vi "edittest read test steps from file.vi"(8 "error in (no error)":errorcluster, 9 "Version":string, 11 "File Refnum In":T2) -> (0 "error out":errorcluster, 2 "Sequence Steps":T1[](array[typedef]), 3 "File Refnum Out":T2)   [LabVIEW 2011]
uses:
  <vilib>/Utility/config.llb/Config Data RefNum.ctl
  server/database/Steps/Step Record.ctl
  <vilib>/Utility/config.llb/Read Key (I32).vi
  <vilib>/Utility/config.llb/Read Key (String).vi
  <vilib>/Utility/config.llb/NI_LVConfig.lvlib
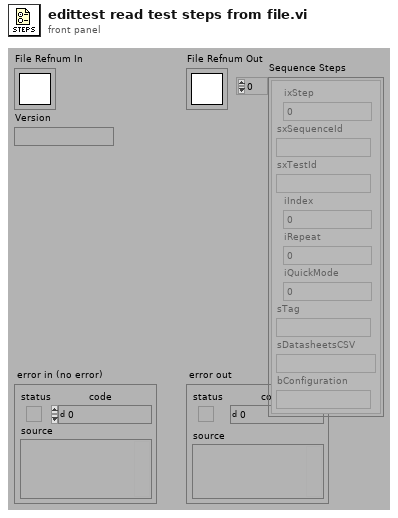
[diagram p1: front panel]
types:
  T1 = typedef "Step Record.ctl" = cluster{"ixStep":i32, "sxSequenceId":string, "sxTestId":string, "iIndex":i32, "iRepeat":i32, "iQuickMode":i32, "sTag":string, "sDatasheetsCSV":string, "bConfiguration":string}
  T2 = typedef "NI_LVConfig.lvlib/Config Data RefNum.ctl" = refnum<k1>
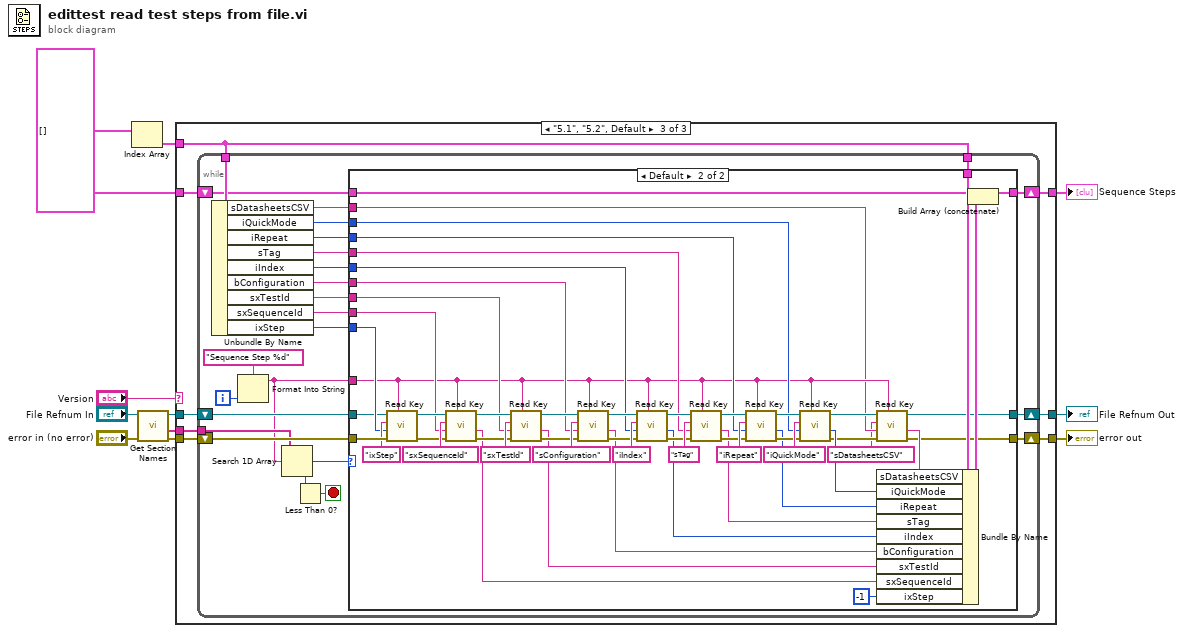
[diagram p0: block diagram]
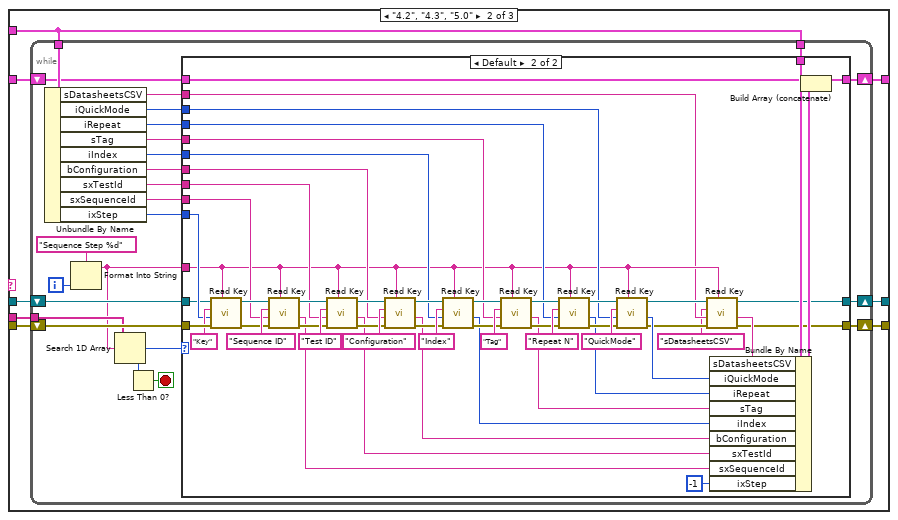
[diagram p3: hidden frame]
diagram:
  w3 = T1[] []
  n1 = Index Array(array=w3) -> (element=w4:T1)  [unwired: 1 in]
  n2 = call <vilib>:"Get Section Names.vi"("error in (no error)"="error in (no error)", "refnum"="File Refnum In") -> ("error out"=w7:errorcluster, "section names"=w5:string[], "refnum out"=w6:T2)  [unwired: 7 out]
  n3 = case shown="\"5.1\", \"5.2\", Default" "Version" {
    tunnel: [w12 w21 w107] -> w11
    tunnel: [w13 w20 w106] -> w10
    tunnel: w7 -> [w12 w19 w105]
    tunnel: w6 -> [w13 w18 w104]
    tunnel: w5 -> [_ w17 w103]
    tunnel: w4 -> [_ w16 w102]
    tunnel: w3 -> [_ w15 w101]
    tunnel: [_ w14 w100] -> w2
    frame "-1.0" {
    }
    frame "4.2", "4.3", "5.0" {
      n4 = while {
        shift-right: [w40] -> w20
        shift-left: w18 -> [w28]
        shift-right: [w41] -> w21
        shift-left: w19 -> [w42]
        tunnel: w16 -> [w39]
        tunnel: w16 -> [w30]
        tunnel: w17 -> [w27]
        shift-right: [w22] -> w14
        shift-left: w15 -> [w23]
        i -> [w43]
        stop <- w24 stop-if-true
        n5 = Unbundle By Name(w39) -> ("sDatasheetsCSV"=w29:string, "iQuickMode"=w31:i32, "iRepeat"=w32:i32, "sTag"=w33:string, "iIndex"=w34:i32, "bConfiguration"=w35:string, "sxTestId"=w36:string, "sxSequenceId"=w37:string, "ixStep"=w38:i32)
        n6 = Format Into String(format string="Sequence Step %d", w43) -> (resulting string=w26:string)  [unwired: 2 in, 1 out]
        n7 = Search 1D Array(1D array=w27, element=w26) -> (index of element=w25:i32)  [unwired: 1 out]
        n8 = Less Than 0?(x=w25) -> (x < 0?=w24:bool)
        n9 = case shown="Default" w25 {
          tunnel: w42 -> [w47 w99]
          tunnel: w26 -> [_ w54]
          tunnel: [w47 w49] -> w41
          tunnel: [w46 w48] -> w40
          tunnel: w38 -> [_ w76]
          tunnel: w37 -> [_ w75]
          tunnel: w36 -> [_ w74]
          tunnel: w35 -> [_ w73]
          tunnel: w34 -> [_ w72]
          tunnel: w33 -> [_ w71]
          tunnel: w32 -> [_ w70]
          tunnel: w31 -> [_ w69]
          tunnel: w30 -> [_ w68]
          tunnel: w29 -> [_ w52]
          tunnel: w28 -> [w46 w60]
          tunnel: w23 -> [w45 w59]
          tunnel: [w45 w57] -> w22
          frame -1 {
          }
          frame Default {
            n10 = call-poly <vilib>:"Read Key.vi"("section"=w54, "error in (no error)"=w99, "default value"=w76, "key"="Key", "refnum"=w60) -> ("error out"=w91:errorcluster, "refnum out"=w82:T2)  [unwired: 5 out]
            n11 = call-poly <vilib>:"Read Key.vi"("section"=w54, "error in (no error)"=w91, "default value"=w75, "key"="Sequence ID", "refnum"=w82) -> ("error out"=w90:errorcluster, "value"=w67:string, "refnum out"=w83:T2)  [unwired: 1 in, 3 out]
            n12 = call-poly <vilib>:"Read Key.vi"("section"=w54, "error in (no error)"=w90, "default value"=w74, "key"="Test ID", "refnum"=w83) -> ("error out"=w77:errorcluster, "value"=w66:string, "refnum out"=w78:T2)  [unwired: 1 in, 3 out]
            n13 = call-poly <vilib>:"Read Key.vi"("section"=w54, "error in (no error)"=w77, "default value"=w73, "key"="Configuration", "refnum"=w78) -> ("error out"=w80:errorcluster, "value"=w65:string, "refnum out"=w79:T2)  [unwired: 1 in, 3 out]
            n14 = call-poly <vilib>:"Read Key.vi"("section"=w54, "error in (no error)"=w80, "default value"=w72, "key"="Index", "refnum"=w79) -> ("error out"=w89:errorcluster, "value"=w64:i32, "refnum out"=w84:T2)  [unwired: 4 out]
            n15 = call-poly <vilib>:"Read Key.vi"("section"=w54, "error in (no error)"=w89, "default value"=w71, "key"="Tag", "refnum"=w84) -> ("error out"=w88:errorcluster, "value"=w63:string, "refnum out"=w85:T2)  [unwired: 1 in, 3 out]
            n16 = call-poly <vilib>:"Read Key.vi"("section"=w54, "error in (no error)"=w88, "default value"=w70, "key"="Repeat N", "refnum"=w85) -> ("error out"=w87:errorcluster, "value"=w62:i32, "refnum out"=w86:T2)  [unwired: 4 out]
            n17 = call-poly <vilib>:"Read Key.vi"("section"=w54, "error in (no error)"=w87, "default value"=w69, "key"="QuickMode", "refnum"=w86) -> ("error out"=w53:errorcluster, "value"=w61:i32, "refnum out"=w55:T2)  [unwired: 4 out]
            n18 = call-poly <vilib>:"Read Key.vi"("section"=w54, "error in (no error)"=w53, "default value"=w52, "key"="sDatasheetsCSV", "refnum"=w55) -> ("error out"=w49:errorcluster, "value"=w50:string, "refnum out"=w48:T2)  [unwired: 1 in, 3 out]
            n19 = Bundle By Name(cluster=w68, "sDatasheetsCSV"=w50, "iQuickMode"=w61, "iRepeat"=w62, "sTag"=w63, "iIndex"=w64, "bConfiguration"=w65, "sxTestId"=w66, "sxSequenceId"=w67, "ixStep"=-1 ("Key")) -> (w58:T1)
            n20 = Build Array (concatenate)(w59, w58) -> (w57:T1[])
          }
        }
      }
    }
    frame "5.1", "5.2", Default {
      n21 = while {
        shift-right: [w126] -> w106
        shift-left: w104 -> [w114]
        shift-right: [w127] -> w107
        shift-left: w105 -> [w128]
        tunnel: w102 -> [w125]
        tunnel: w102 -> [w116]
        tunnel: w103 -> [w113]
        shift-right: [w108] -> w100
        shift-left: w101 -> [w109]
        i -> [w129]
        stop <- w110 stop-if-true
        n22 = Unbundle By Name(w125) -> ("sDatasheetsCSV"=w115:string, "iQuickMode"=w117:i32, "iRepeat"=w118:i32, "sTag"=w119:string, "iIndex"=w120:i32, "bConfiguration"=w121:string, "sxTestId"=w122:string, "sxSequenceId"=w123:string, "ixStep"=w124:i32)
        n23 = Format Into String(format string="Sequence Step %d", w129) -> (resulting string=w112:string)  [unwired: 2 in, 1 out]
        n24 = Search 1D Array(1D array=w113, element=w112) -> (index of element=w111:i32)  [unwired: 1 out]
        n25 = Less Than 0?(x=w111) -> (x < 0?=w110:bool)
        n26 = case shown="Default" w111 {
          tunnel: w128 -> [w133 w185]
          tunnel: w112 -> [_ w140]
          tunnel: [w133 w135] -> w127
          tunnel: [w132 w134] -> w126
          tunnel: w124 -> [_ w162]
          tunnel: w123 -> [_ w161]
          tunnel: w122 -> [_ w160]
          tunnel: w121 -> [_ w159]
          tunnel: w120 -> [_ w158]
          tunnel: w119 -> [_ w157]
          tunnel: w118 -> [_ w156]
          tunnel: w117 -> [_ w155]
          tunnel: w116 -> [_ w154]
          tunnel: w115 -> [_ w138]
          tunnel: w114 -> [w132 w146]
          tunnel: w109 -> [w131 w145]
          tunnel: [w131 w143] -> w108
          frame -1 {
          }
          frame Default {
            n27 = call-poly <vilib>:"Read Key.vi"("section"=w140, "error in (no error)"=w185, "default value"=w162, "key"="ixStep", "refnum"=w146) -> ("error out"=w177:errorcluster, "refnum out"=w168:T2)  [unwired: 5 out]
            n28 = call-poly <vilib>:"Read Key.vi"("section"=w140, "error in (no error)"=w177, "default value"=w161, "key"="sxSequenceId", "refnum"=w168) -> ("error out"=w176:errorcluster, "value"=w153:string, "refnum out"=w169:T2)  [unwired: 1 in, 3 out]
            n29 = call-poly <vilib>:"Read Key.vi"("section"=w140, "error in (no error)"=w176, "default value"=w160, "key"="sxTestId", "refnum"=w169) -> ("error out"=w163:errorcluster, "value"=w152:string, "refnum out"=w164:T2)  [unwired: 1 in, 3 out]
            n30 = call-poly <vilib>:"Read Key.vi"("section"=w140, "error in (no error)"=w163, "default value"=w159, "key"="sConfiguration", "refnum"=w164) -> ("error out"=w166:errorcluster, "value"=w151:string, "refnum out"=w165:T2)  [unwired: 1 in, 3 out]
            n31 = call-poly <vilib>:"Read Key.vi"("section"=w140, "error in (no error)"=w166, "default value"=w158, "key"="iIndex", "refnum"=w165) -> ("error out"=w175:errorcluster, "value"=w150:i32, "refnum out"=w170:T2)  [unwired: 4 out]
            n32 = call-poly <vilib>:"Read Key.vi"("section"=w140, "error in (no error)"=w175, "default value"=w157, "key"="sTag", "refnum"=w170) -> ("error out"=w174:errorcluster, "value"=w149:string, "refnum out"=w171:T2)  [unwired: 1 in, 3 out]
            n33 = call-poly <vilib>:"Read Key.vi"("section"=w140, "error in (no error)"=w174, "default value"=w156, "key"="iRepeat", "refnum"=w171) -> ("error out"=w173:errorcluster, "value"=w148:i32, "refnum out"=w172:T2)  [unwired: 4 out]
            n34 = call-poly <vilib>:"Read Key.vi"("section"=w140, "error in (no error)"=w173, "default value"=w155, "key"="iQuickMode", "refnum"=w172) -> ("error out"=w139:errorcluster, "value"=w147:i32, "refnum out"=w141:T2)  [unwired: 4 out]
            n35 = call-poly <vilib>:"Read Key.vi"("section"=w140, "error in (no error)"=w139, "default value"=w138, "key"="sDatasheetsCSV", "refnum"=w141) -> ("error out"=w135:errorcluster, "value"=w136:string, "refnum out"=w134:T2)  [unwired: 1 in, 3 out]
            n36 = Bundle By Name(cluster=w154, "sDatasheetsCSV"=w136, "iQuickMode"=w147, "iRepeat"=w148, "sTag"=w149, "iIndex"=w150, "bConfiguration"=w151, "sxTestId"=w152, "sxSequenceId"=w153, "ixStep"=-1 ("Key")) -> (w144:T1)
            n37 = Build Array (concatenate)(w145, w144) -> (w143:T1[])
          }
        }
      }
    }
  }
  "error out" <- w11
  "File Refnum Out" <- w10
  "Sequence Steps" <- w2
